vi "GetData.vi"(8 "error in (no error)":errorcluster, 9 "SequenceNumber":u32, 10 "address":u32, 11 "connection ID":refnum<k16>) -> (0 "error out":errorcluster, 1 "SequenceNumber out":i32, 2 "Address out":u32, 3 "connection ID out":refnum<k16>, 5 "data out":string)   [LabVIEW 2009]
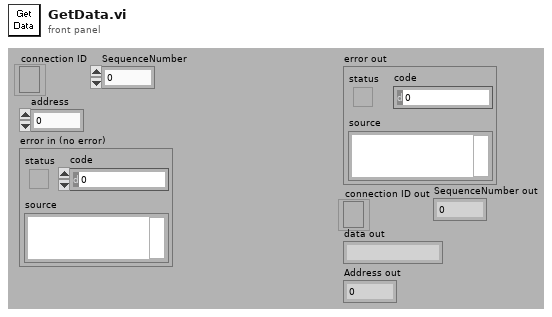
[diagram p1: front panel]
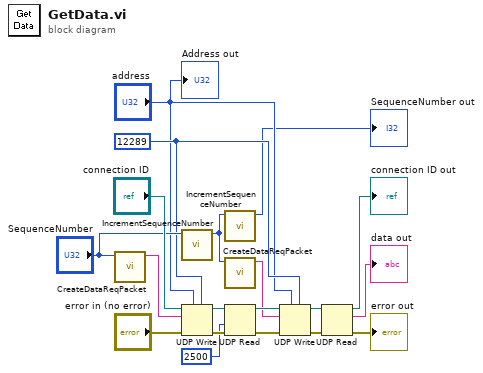
[diagram p0: block diagram]
diagram:
  w6 = u16 12289 ("port or service name")
  n1 = call "CreateDataReqPacket.vi"("SequenceNumber"="SequenceNumber") -> ("DataReqPacket"=w18:string)  [unwired: 6 in]
  n2 = call "IncrementSequenceNumber.vi"("In"="SequenceNumber") -> ("Out"=w2:i32)  [unwired: 10 in]
  n3 = UDP Write(address="address", port or service name=w6, connection ID="connection ID", data in=w18, 8:"error in (no error)") -> (error out=w13:errorcluster, 3:w16:refnum<k16>)  [unwired: 1 in]
  n4 = call "IncrementSequenceNumber.vi"("In"=w2) -> ("Out"=→"SequenceNumber out":i32)  [unwired: 10 in]
  n5 = call "CreateDataReqPacket.vi"("SequenceNumber"=w2) -> ("DataReqPacket"=w7:string)  [unwired: 6 in]
  n6 = UDP Read(connection ID=w16, timeout ms (25000)=2500, 8:w13) -> (error out=w12:errorcluster, 3:w15:refnum<k16>)  [unwired: 1 in, 3 out]
  n7 = UDP Write(address="address", port or service name=w6, connection ID=w15, data in=w7, 8:w12) -> (error out=w11:errorcluster, 3:w14:refnum<k16>)  [unwired: 1 in]
  n8 = UDP Read(connection ID=w14, 8:w11) -> (data out=→"data out":string, error out=→"error out":errorcluster, 3:→"connection ID out":refnum<k16>)  [unwired: 2 in, 2 out]
  "Address out" <- "address"
